vi "SUSLabPI.vi"() -> ()   [LabVIEW 2020]
uses:
  <vilib>/Utility/file.llb/Read Delimited Spreadsheet (DBL).vi
panel:
  out "u4":dbl=128.56052631578947
  out "is":dbl
  out "output variable 3":dbl=38.56422452708354
  in  "input variable":dbl format="%#_13g"
  out "output variable 2":dbl=0.0012259744206915002
  in  "isNoise":bool
  out "output variable":i32
  out "u 3":dbl
  in  "u 2":dbl(knob) scale=0.0..100.0
  in  "Td":dbl=14.14644
  in  "u":dbl(knob) scale=0.0..100.0
  in  "h":dbl=1.0 format="%#_13g"
  out "Cr":dbl=38.56422452708354
  out "e":dbl=0.0012259744206915002
  in  "Tzad":dbl=70.0
  in  "Ti":dbl=58.9435
  in  "k":dbl=70.7322
  out "ybez":dbl=69.99877402557931
  out "Waveform Graph":dbl[][](graph)
  out "all rows":dbl[][](array[numeric])
  out "y":dbl=70.00051853165213
  in  "Thin":dbl=19.0
  in  "F":dbl=1.3
  in  "Delay":u32=10
  out "U":dbl=38.56422452708354
  in  "stop":bool
  out "Wykers":cluster{"Xwy":dbl, "Xwy":dbl}(graph)
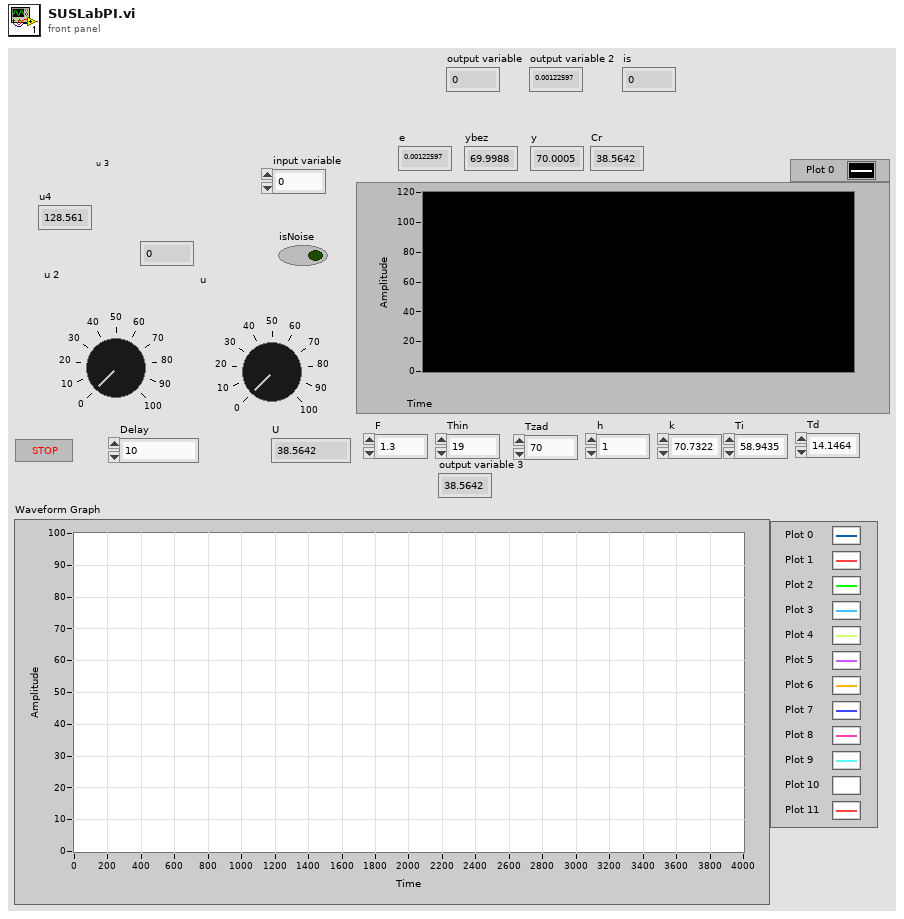
[diagram p1: front panel]
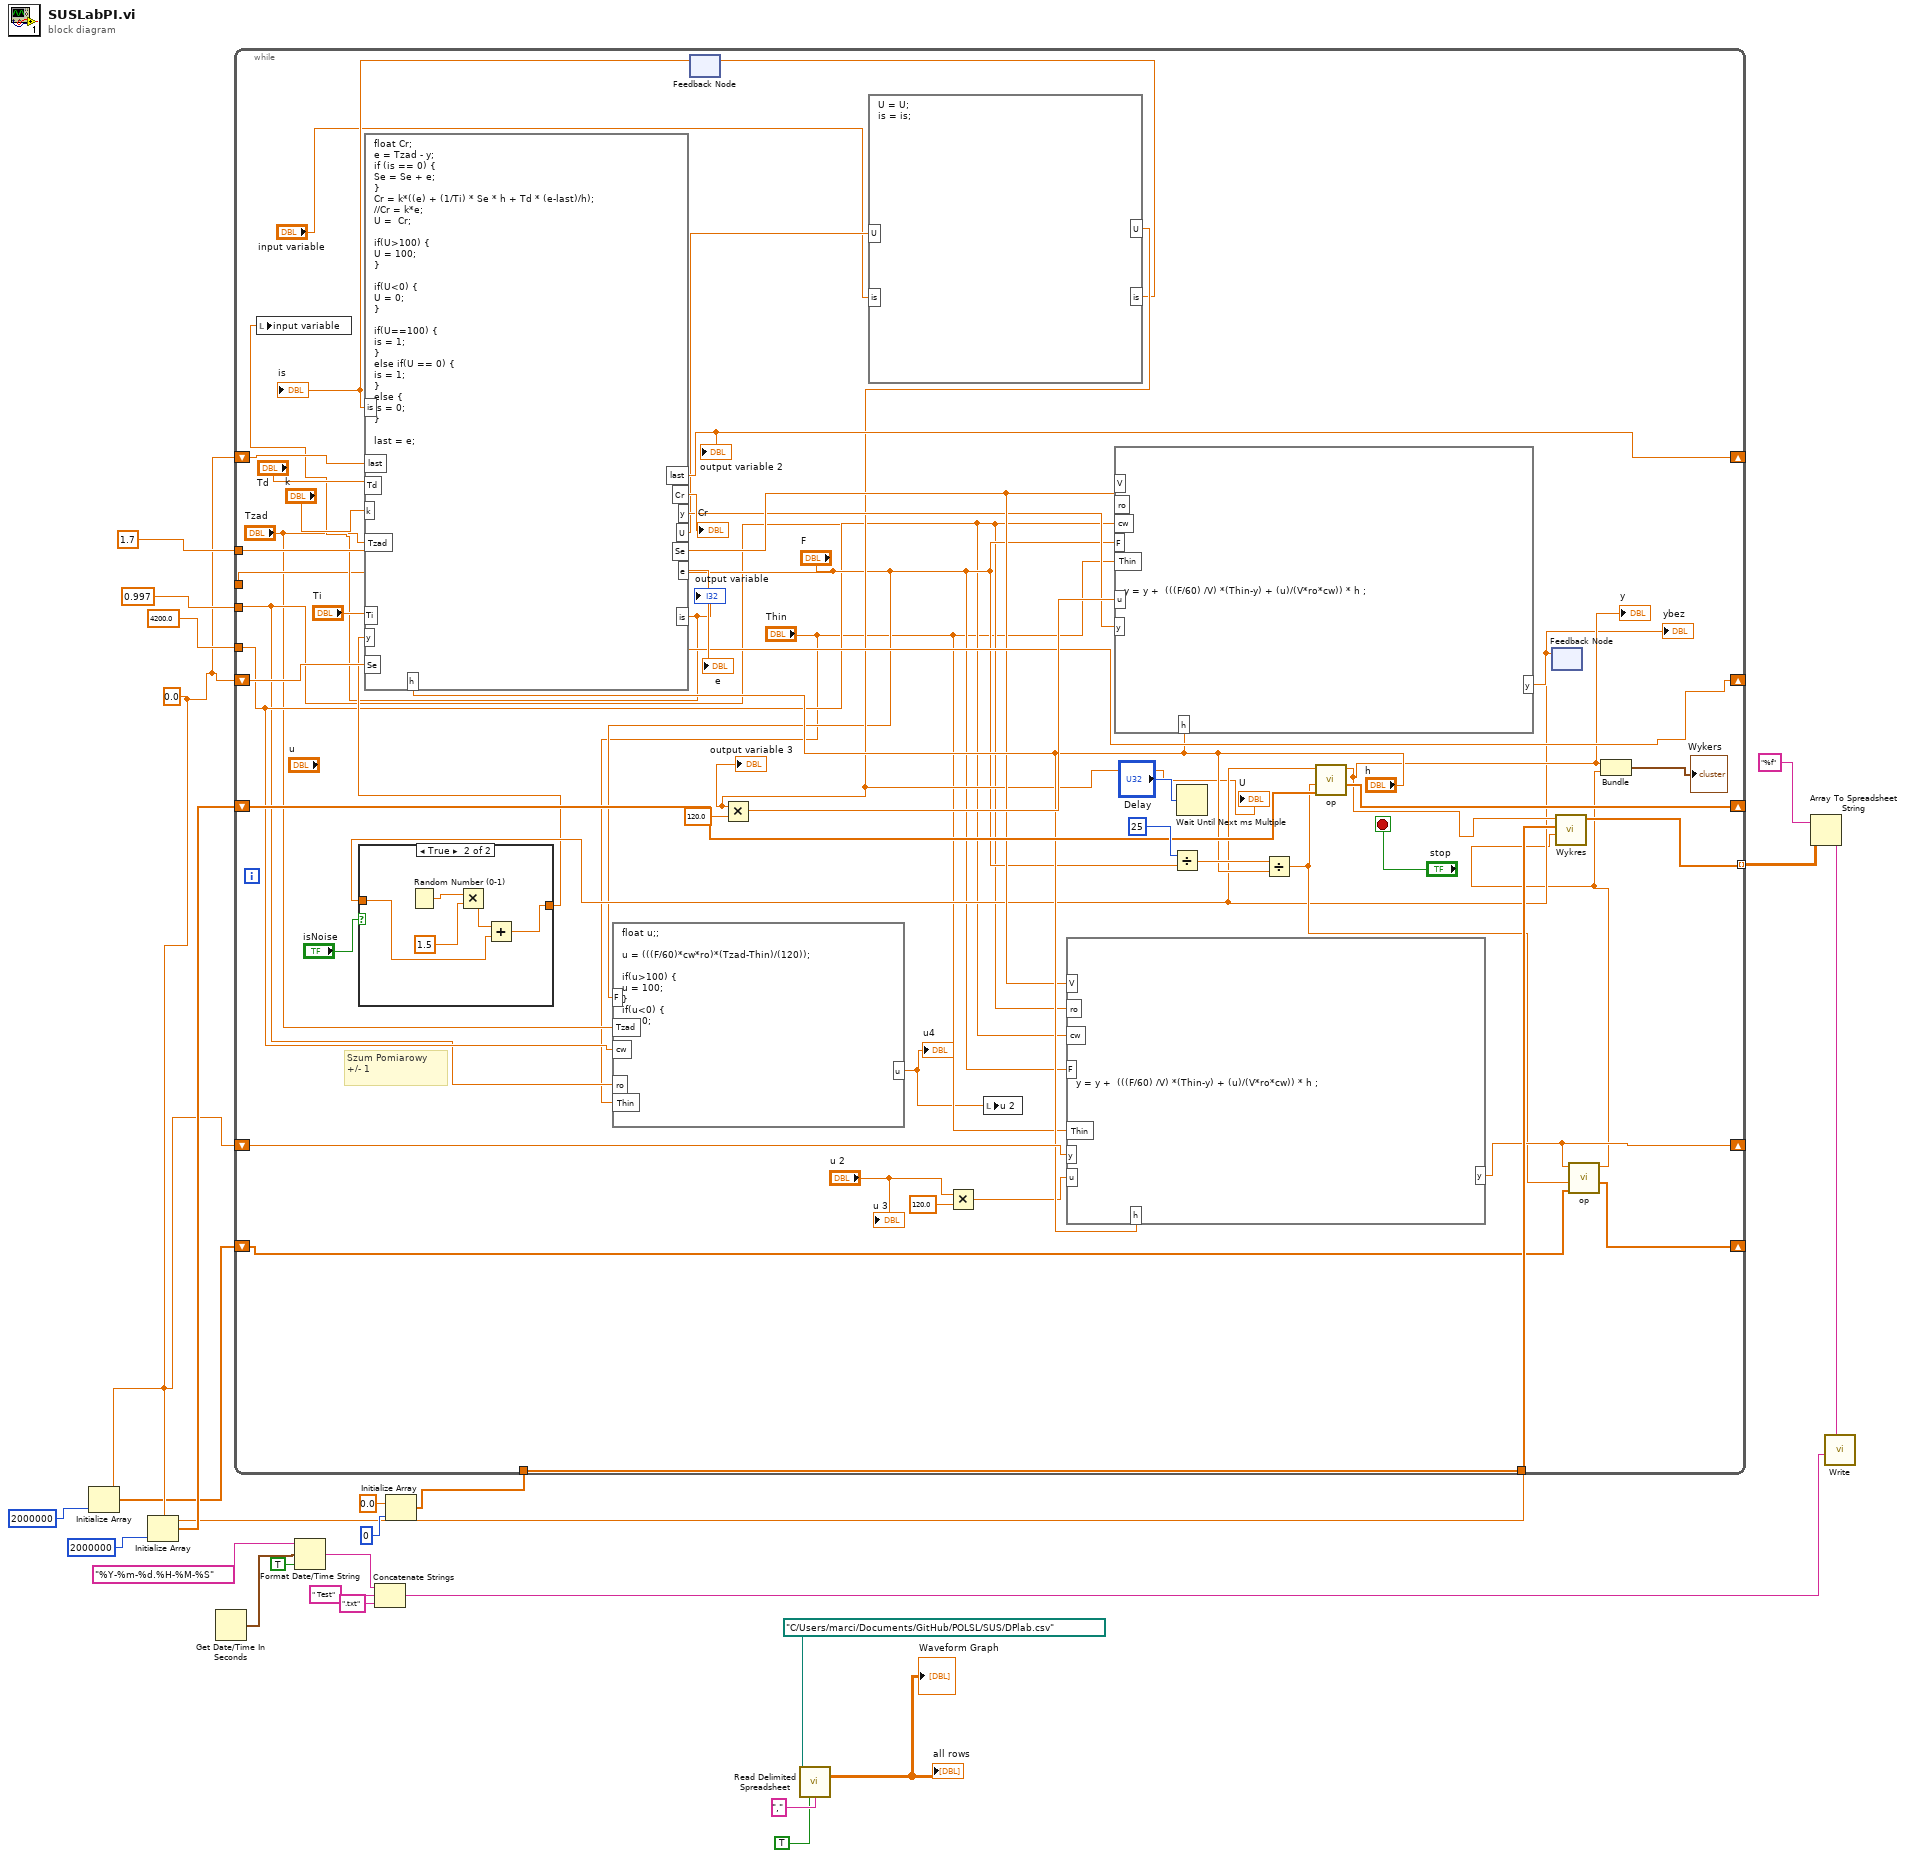
[diagram p0: block diagram]
diagram:
  w2 = 0.0
  n1 = Initialize Array(w2, 2000000 ("dimension size")) -> (w1:dbl[])
  n2 = Initialize Array(w2, 2000000 ("dimension size")) -> (w5:dbl[])
  n3 = Get Date/Time In Seconds() -> (seconds since 1Jan1904=w17:timestamp)
  n4 = Format Date/Time String(time format string (%c)="%Y-%m-%d.%H-%M-%S", seconds (now)=w17, UTC format=TRUE) -> (date/time string=w15:string)
  n5 = Concatenate Strings(w15, " Test" ("string"), ".txt" ("string")) -> (w12:string)
  n6 = Initialize Array(0.0 ("element"), 0 ("dimension size")) -> (w4:dbl[])
  n7 = while {
    tunnel: 1.7 ("V") -> [w45]
    tunnel: 0.997 ("ro") -> [w32]
    tunnel: 4200.0 ("cw") -> [w33]
    tunnel: [w47] -> w11 mode=indexing
    tunnel: w4 -> [w73]
    tunnel: ["F"] -> _
    shift-right: [w70] -> _
    shift-left: w5 -> [w71]
    tunnel: w2 -> [_]
    shift-right: [w59] -> _
    shift-left: w2 -> [w60]
    shift-right: [w56] -> _
    shift-left: w2 -> [w57]
    shift-right: [w53] -> _
    shift-left: w2 -> [w55]
    shift-right: [w50] -> _
    shift-left: w1 -> [w49]
    stop <- "stop" stop-if-true
    # "Szum Pomiarowy\n+/- 1"
    n8 = formula code="float u;;\n\nu = (((F/60)*cw*ro)*(Tzad-Thin)/(120));\n\nif(u>100) {\nu = 100;\n}\nif(u<0) {\nu = 0;\n}"("F"="F", "Tzad"="Tzad", "cw"=w33, "ro"=w32, "Thin"="Thin") -> ("u"=w28:dbl)
    "u4" <- w28
    n9 = feedback #1() -> (w37:dbl)  [unwired: 1 in]
    "is" <- w37
    n10 = Multiply(x="u 2", y=120.0) -> (x*y=w29:dbl)
    n11 = local write "u 2"(w28) -> ()
    n12 = formula code="y = y +  (((F/60) /V) *(Thin-y) + (u)/(V*ro*cw)) * h ;"("u"=w29, "y"=w55, "Thin"="Thin", "F"="F", "cw"=w33, "ro"=w32, "V"=w45, "h"="h") -> ("y"=w53:dbl)
    n13 = Divide(x=25, y="F") -> (x/y=w52:dbl)
    n14 = Wait Until Next ms Multiple(millisecond multiple="Delay") -> ()  [unwired: 1 out]
    n15 = Divide(x=w52, y="h") -> (x/y=w51:dbl)
    n16 = feedback #2() -> (w42:dbl)  [unwired: 1 in]
    "ybez" <- w42
    n17 = case shown="True" "isNoise" {
      tunnel: w42 -> [w75 w78]
      tunnel: [w75 w76] -> w41
      frame False {
      }
      frame True {
        n18 = Random Number (0-1)() -> (number: 0 to 1=w80:dbl)
        n19 = Multiply(x=w80, y=1.5) -> (x*y=w77:dbl)
        n20 = Add(x=w77, y=w78) -> (x+y=w76:dbl)
      }
    }
    n21 = formula code="float Cr;\ne = Tzad - y;\nif (is == 0) {\nSe = Se + e;\n}\nCr = k*((e) + (1/Ti) * Se * h + Td * (e-last)/h);\n//Cr = k*e;\nU =  Cr;\n\nif(U>100) {\nU = 100;\n}\n\nif(U<0) {\nU = 0;\n}\n\nif(U==100) {\nis = 1;\n}\nelse if(U == 0) {\nis = 1;\n}\nelse {\nis = 0;\n}\n\nlast = e;"("k"="k", "Ti"="Ti", "Se"=w60, "y"=w41, "Tzad"="Tzad", "h"="h", "Td"="Td", "last"=w57, "is"=w37) -> ("e"=→"e":dbl, "y"=w44:dbl, "U"=w40:dbl, "Cr"=→"Cr":dbl, "Se"=w59:dbl, "last"=w56:dbl, "is"=w36:dbl)
    "output variable" <- w36
    "output variable 2" <- w56
    n22 = local write "input variable"(w36) -> ()
    n23 = formula code="U = U;\nis = is;"("U"=w40, "is"="input variable") -> ("U"=w39:dbl, "is"=w38:dbl)
    "U" <- w39
    "output variable 3" <- w39
    n24 = feedback-in #1(w38) -> ()
    n25 = Multiply(x=w39, y=120.0) -> (x*y=w63:dbl)
    n26 = formula code="y = y +  (((F/60) /V) *(Thin-y) + (u)/(V*ro*cw)) * h ;"("u"=w63, "y"=w44, "Thin"="Thin", "F"="F", "cw"=w33, "ro"=w32, "V"=w45, "h"="h") -> ("y"=w61:dbl)
    n27 = call "op.vi"("initialized array"=w71, "delay"=w51, "Xwe"=w42) -> ("s? t:f"=w70:dbl[], "Xwy"=w46:dbl)  [unwired: 7 in]
    "y" <- w46
    n28 = feedback-in #2(w61) -> ()
    n29 = call "op.vi"("initialized array"=w49, "delay"=w51, "Xwe"=w53) -> ("s? t:f"=w50:dbl[], "Xwy"=w26:dbl)  [unwired: 7 in]
    n30 = call "Wykres.vi"("new element/subarray"=w26, "initialized array"=w73, "Y"=w46) -> ("output array"=w47:dbl[])  [unwired: 8 in]
    n31 = Bundle("Xwy"=w46, "Xwy"=w26) -> (→"Wykers":cluster{"Xwy":dbl, "Xwy":dbl})  [unwired: 1 in]
    "u 3" <- "u 2"
  }
  n32 = call-poly <vilib>:"Read Delimited Spreadsheet.vi"("file path (dialog if empty)"=path "C:/Users/marci/Documents/GitHub/POLSL/SUS/DPlab.csv", "transpose? (F)"=TRUE, "delimiter (\\t)"="," ("delimiter (\\t)")) -> ("all rows"=→"all rows" →"Waveform Graph":dbl[][])  [unwired: 7 in, 5 out]
  n33 = Array To Spreadsheet String(array=w11, 3:"%f" ("format string")) -> (spreadsheet string=w9:string)  [unwired: 1 in]
  n34 = call "Write.vi"("File Name"=w12, "text"=w9) -> ()  [unwired: 9 in, 1 out]
